vi "Data Check DC Rectifier Settings.vi"(9 "String":string, 10 "Coords":T1, 11 "MulticolumnListbox in":refnum<vi>) -> (0 "error out":errorcluster, 3 "reference out":refnum<vi>)   [LabVIEW 2019]
uses:
  <vilib>/Utility/miscctls.llb/LVRowAndColumnTypeDef.ctl
  <vilib>/regexp/Match Regular Expression.xnode
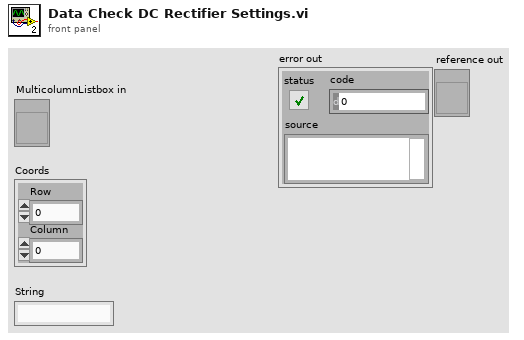
[diagram p1: front panel]
types:
  T1 = typedef "LVRowAndColumnTypeDef.ctl" = cluster{"Row":i32, "Column":i32}
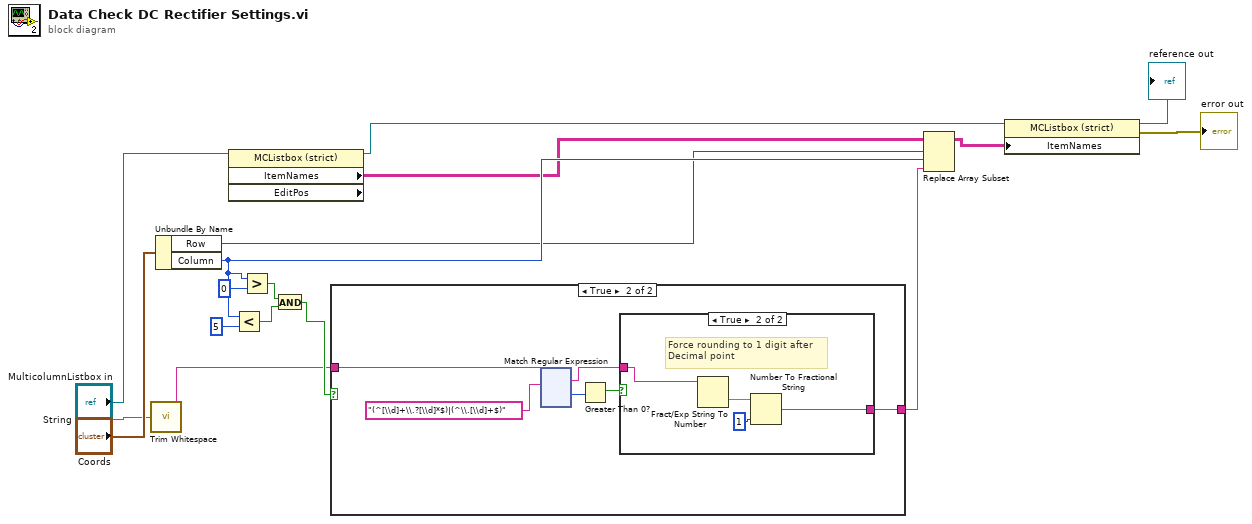
[diagram p0: block diagram]
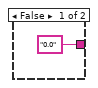
[diagram p3: hidden frame]
diagram:
  n1 = call <vilib>:"Trim Whitespace.vi"("string"="String") -> ("trimmed string"=w4:string)  [unwired: 1 in]
  n2 = Unbundle By Name("Coords") -> ("Row"=w11:i32, "Column"=w13:i32)
  n3 = property class="MCListbox (strict)" props=["ItemNames", "EditPos"](reference="MulticolumnListbox in") -> (reference out=w7:refnum<vi>, "ItemNames"=w8:string[][])  [unwired: 1 in, 2 out]
  n4 = Less?(x=w13, y=5) -> (x < y?=w16:bool)
  n5 = Greater?(x=w13, y=0) -> (0:w15:bool)
  n6 = And(x=w15, y=w16) -> (x .and. y?=w17:bool)
  n7 = case shown="True" w17 {
    tunnel: w4 -> [w18 w24]
    tunnel: [w18 w19] -> w10
    frame False {
    }
    frame True {
      n8 = xnode "Match Regular Expression"("input string"=w24, "regular expression"="(^[\\d]+\\.?[\\d]*$)|(^\\.[\\d]+$)") -> ("whole match"=w20:string, "offset past match"=w22:i32)  [unwired: 4 in, 3 out]
      n9 = Greater Than 0?(x=w22) -> (x > 0?=w21:bool)
      n10 = case shown="True" w21 {
        tunnel: w20 -> [_ w29]
        tunnel: ["0.0" w26] -> w19
        frame False {
        }
        frame True {
          # "Force rounding to 1 digit after\nDecimal point"
          n11 = Fract/Exp String To Number(string=w29) -> (number=w28:dbl)  [unwired: 3 in, 1 out]
          n12 = Number To Fractional String(number=w28, precision (6)=i16 1) -> (F-format string=w26:string)  [unwired: 2 in]
        }
      }
    }
  }
  n13 = Replace Array Subset(array=w8, new element=w10, index (row)=w11, index (col)=w13) -> (w9:string[][])
  n14 = property class="MCListbox (strict)"(reference=w7, "ItemNames"=w9) -> (reference out=→"reference out":refnum<vi>, error out=→"error out":errorcluster)  [unwired: 1 in]
